vi "Match_Style_Classes_and_Names.vi"() -> ()   [LabVIEW 2025]
uses:
  <vilib>/Utility/error.llb/Trim Whitespace One-Sided.vi
panel:
  out "spreadsheet string":string
  out "Array":string[][](array[string])
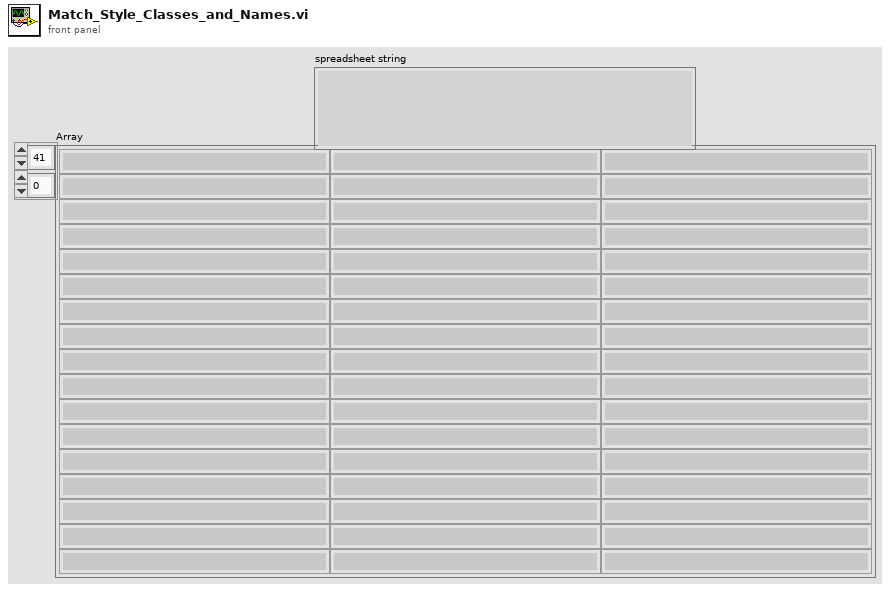
[diagram p1: front panel]
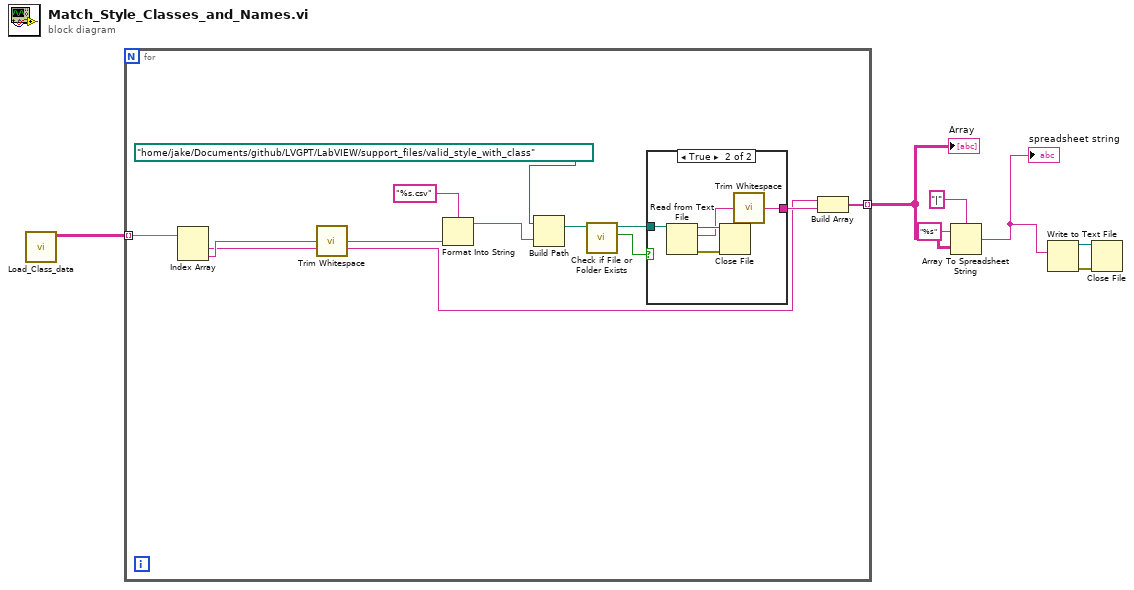
[diagram p0: block diagram]
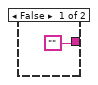
[diagram p2: hidden frame]
diagram:
  n1 = call "Load_Class_data.vi"() -> ("Styles and IDs"=w7:string[][])  [unwired: 10 in, 1 out]
  n2 = for {
    tunnel: w7 -> [w19] mode=indexing
    tunnel: [w9] -> w6 mode=indexing
    n3 = Index Array(array=w19) -> (element #1=w10:string, element #2=w17:string)  [unwired: 2 in]
    n4 = call <vilib>:"Trim Whitespace.vi"("string"=w17) -> ("trimmed string"=w8:string)  [unwired: 1 in]
    n5 = Format Into String(format string="%s.csv", w8) -> (resulting string=w16:string)  [unwired: 2 in, 1 out]
    n6 = Build Path(base path=path "/home/jake/Documents/github/LVGPT/LabVIEW/support_files/valid_style_with_class", name or relative path=w16) -> (appended path=w14:path)
    n7 = call <vilib>:"Check if File or Folder Exists.vi"("path"=w14) -> ("file or folder exists?"=w13:bool, "dup path"=w12:path)  [unwired: 8 in, 1 out]
    n8 = case shown="True" w13 {
      tunnel: w12 -> [_ w25]
      tunnel: ["" w21] -> w11
      frame False {
      }
      frame True {
        n9 = Read from Text File(file (use dialog)=w25) -> (refnum out=w23:refnum<file>, text=w22:string, error out=w24:errorcluster)  [unwired: 3 in, 1 out]
        n10 = Close File(refnum=w23, error in=w24) -> ()  [unwired: 2 out]
        n11 = call <vilib>:"Trim Whitespace.vi"("string"=w22) -> ("trimmed string"=w21:string)  [unwired: 1 in]
      }
    }
    n12 = Build Array(w10, w11) -> (w9:string[])
  }
  "Array" <- w6
  n13 = Array To Spreadsheet String(delimiter (Tab)="|", array=w6, 3:"%s" ("format string")) -> (spreadsheet string=w3:string)
  "spreadsheet string" <- w3
  n14 = Write to Text File(text=w3) -> (refnum out=w1:refnum<file>, error out=w2:errorcluster)  [unwired: 3 in, 1 out]
  n15 = Close File(refnum=w1, error in=w2) -> ()  [unwired: 2 out]
